vi "CTRE_ErrorHandle.vi"(8 "error in":errorcluster, 10 "origin":string, 11 "code":i32) -> (0 "error out":errorcluster)   [LabVIEW 2016]
uses:
  <vilib>/Utility/error.llb/whitespace.ctl
  Controls/DriverLib.ctl
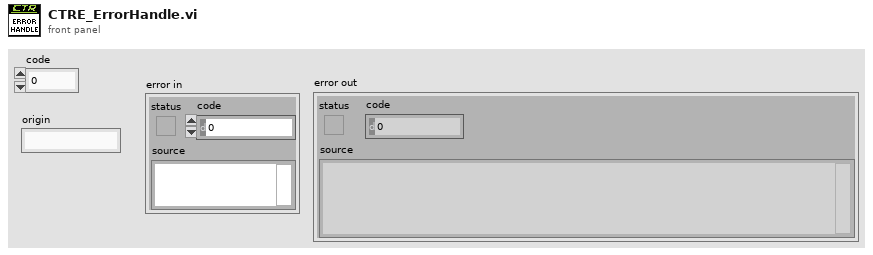
[diagram p1: front panel]
types:
  T1 = typedef "DriverLib.ctl" = path
  T2 = typedef "whitespace.ctl" = u16
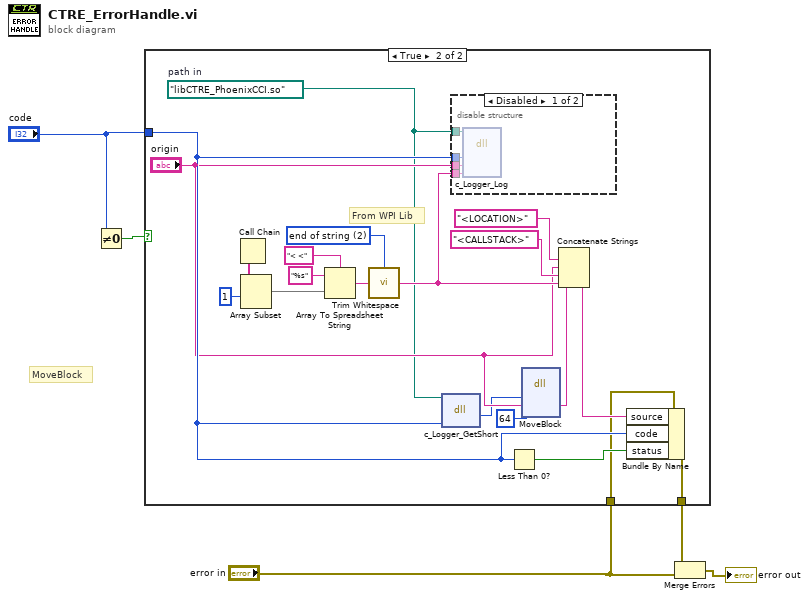
[diagram p0: block diagram]
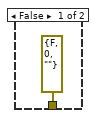
[diagram p2: hidden frame]
diagram:
  # "MoveBlock"
  n1 = Not Equal To 0?(x="code") -> (x != 0?=w4:bool)
  n2 = case shown="True" w4 {
    tunnel: "code" -> [_ w15]
    tunnel: [errorcluster {"status"=FALSE, "code"=0, "source"=""} ("error in") w13] -> w2
    tunnel: "error in" -> [_ w12]
    frame False {
    }
    frame True {
      w7 = T1 path "libCTRE_PhoenixCCI.so"  # path in
      w23 = T2 2 items=["both", "start of string", "end of string"] ("location (both)")
      # "From WPI Lib"
      n3 = Call Chain() -> (call chain=w19:string[])
      n4 = Array Subset(array=w19, index=1) -> (w20:string[])  [unwired: 1 in]
      n5 = Array To Spreadsheet String(delimiter (Tab)="< <", array=w20, 3:"%s" ("format string")) -> (spreadsheet string=w24:string)
      n6 = call <vilib>:"Trim Whitespace.vi"("string"=w24, "location (both)"=w23) -> ("trimmed string"=w17:string)
      n7 = dll-call lib="?" fn="c_Logger_GetShort"(path in=w7, "CTRCode"=w15) -> ("return type"=w8:i64)  [unwired: 3 in, 2 out]
      n8 = disable-structure shown="Disabled" {
        disable-tunnel: w17 -> [w30 _]
        disable-tunnel: w15 -> [w29 _]
        disable-tunnel: "origin" -> [w28 _]
        disable-tunnel: w7 -> [w27 _]
        frame Disabled {
          n9 = dll-call lib="?" fn="c_Logger_Log" label="Call Library Function Node"(path in=w27, "CTRCode"=w29, "origin"=w28, "stacktrace"=w30) -> ()  [unwired: 6 in, 2 out]
        }
        frame Enabled {
        }
      }
      n10 = Less Than 0?(x=w15) -> (x < 0?=w16:bool)
      n11 = dll-call lib="LabVIEW" fn="MoveBlock"("Address (Pointer)"=w8, "Destination"="origin", "Size"=64) -> ("Destination"=w10:string)  [unwired: 6 in, 2 out]
      n12 = Concatenate Strings(w10, "<LOCATION>" ("string"), "origin", "<CALLSTACK>" ("string"), w17) -> (w14:string)
      n13 = Bundle By Name(cluster=w12, "source"=w14, "code"=w15, "status"=w16) -> (w13:errorcluster)
    }
  }
  n14 = Merge Errors(w2, "error in") -> (→"error out":errorcluster)
